vi "MonitorRheometer.vi"() -> ()   [LabVIEW 2017]
uses:
  ImageAcquisitionProgram/ImageAcquisitionLibrary/Acquisition/AcquireData.ctl
  ImageAcquisitionProgram/ImageAcquisitionLibrary/GlobalFrontPanelReferences.vi
  CoilsControl/FrontPanelReferences.vi
  AODControl/AODGlobals.vi
  AODControl/MessageQueue/QueueOperations/Enqueue Message (Single).vi
  ImageAcquisitionProgram/ImageAcquisitionLibrary/ImageAcquisitionLibrary.lvlib
  <vilib>/Analysis/NI_AAL_Geometry.lvlib
  <vilib>/gmath/NI_Gmath.lvlib
  CoilsControl/WaveformGenerator.lvlib
  AODControl/AODControl.lvlib
  AODControl/MessageQueue/MessageQueue.lvlib
panel:
  out "size(s)":i32
  out "r":dbl format="%.2f"
  out "logical OR":bool
  in  "stop":bool
  out "Tracking Data.Positions":dbl[][](array[numeric])
  out "XY Graph":cluster{dbl[], dbl[]}[](graph)
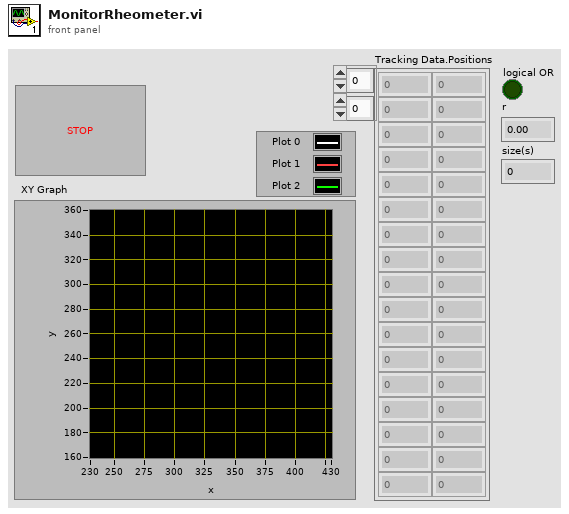
[diagram p1: front panel]
types:
  T1 = typedef "ImageAcquisitionLibrary.lvlib/AcquireData.ctl" = cluster{"Frame Data":cluster{"Image":u32[][], "Timestamp":timestamp, "Image Type":T2, "Dropped Frames":u32}, "Tracking Data":cluster{"Positions":dbl[][], "Timestamp":timestamp}, "Tracked?":bool}
  T2 = typedef "Image Type" = u32
  T3 = typedef "ImageAcquisitionLibrary.lvlib/References.ctl" = cluster{"Acquire":refnum<vi>, "Rec":refnum<vi>, "Tracking":refnum<vi>, "Settings":refnum<vi>, "Stop":refnum<vi>, "Initialized?":bool, "ImDisplay":refnum<vi>}
  T4 = typedef "WaveformGenerator.lvlib/WaveformGeneratorInterfaceRef.ctl" = cluster{"Waveform X":refnum<vi>, "Waveform Y":refnum<vi>, "Waveform Z":refnum<vi>, "Amplitude X":refnum<vi>, "Amplitude Y":refnum<vi>, "Amplitude Z":refnum<vi>, "Frequency X":refnum<vi>, "Frequency Y":refnum<vi>, "Frequency Z":refnum<vi>, "Phase X":refnum<vi>, "Phase Y":refnum<vi>, "Phase Z":refnum<vi>, "Offset X":refnum<vi>, "Offset Y":refnum<vi>, "Offset Z":refnum<vi>, "Stop":refnum<vi>, "On/Off":refnum<vi>, "Field^2":refnum<vi>}
  T5 = typedef "AODControl.lvlib/MessageQueue.lvlib/All Message Queues.ctl" = cluster{" AOD Interface":refnum<queue>}
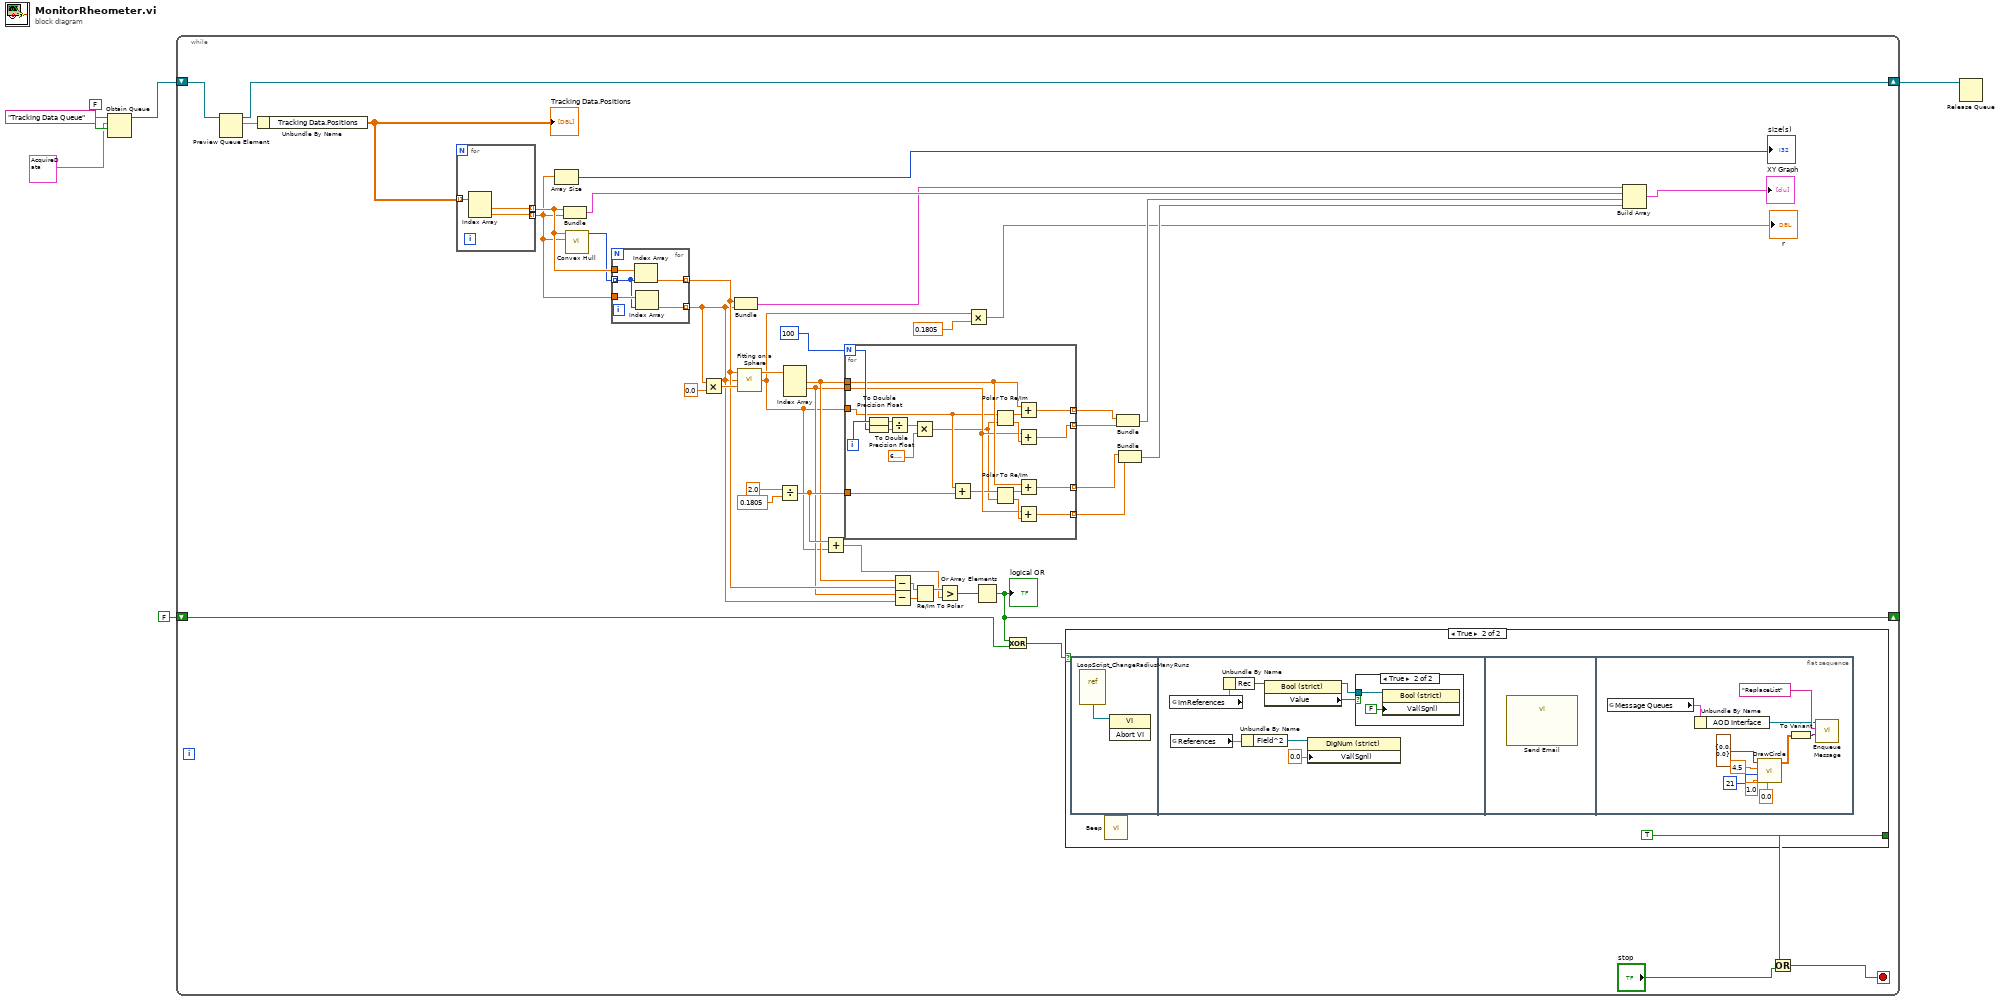
[diagram p0: block diagram]
diagram:
  n1 = Obtain Queue(name (unnamed)="Tracking Data Queue", element data type=T1 {"Frame Data"={"Image"=[], "Timestamp"=timestamp(0 s since 1904-01-01), "Image Type"=0, "Dropped Frames"=0}, "Tracking Data"={"Positions"=[], "Timestamp"=timestamp(0 s since 1904-01-01)}, "Tracked?"=FALSE} ("Acquired Data"), create if not found? (T)=FALSE) -> (queue out=w4:refnum<queue>)  [unwired: 2 in, 2 out]
  n2 = while {
    shift-right: [w45] -> w2
    shift-left: w4 -> [w48]
    shift-right: [w17] -> _
    shift-left: FALSE -> [w16]
    stop <- w9 stop-if-true
    n3 = Preview Queue Element(queue=w48) -> (queue out=w45:refnum<queue>, element=w47:T1)  [unwired: 2 in, 2 out]
    n4 = Unbundle By Name(w47) -> ("Tracking Data.Positions"=w46:dbl[][])
    "Tracking Data.Positions" <- w46
    n5 = for {
      tunnel: w46 -> [w97] mode=indexing
      tunnel: [w96] -> w44 mode=indexing
      tunnel: [w95] -> w11 mode=indexing
      n6 = Index Array(array=w97) -> (element #1=w96:dbl, element #2=w95:dbl)  [unwired: 2 in]
    }
    n7 = Array Size(array=w11) -> (size(s)=→"size(s)":i32)
    n8 = Bundle(w44, w11) -> (w41:cluster{dbl[], dbl[]})  [unwired: 1 in]
    n9 = call <vilib>:"Convex Hull.vi"("Y"=w11, "X"=w44) -> ("Convex Hull"=w43:i32[])  [unwired: 8 in, 1 out]
    n10 = for {
      tunnel: w44 -> [w94]
      tunnel: w11 -> [w93]
      tunnel: w43 -> [w92] mode=indexing
      tunnel: [w91] -> w19 mode=indexing
      tunnel: [w90] -> w21 mode=indexing
      n11 = Index Array(array=w94, index=w92) -> (element=w90:dbl)
      n12 = Index Array(array=w93, index=w92) -> (element=w91:dbl)
    }
    n13 = Multiply(x=w19, y=0.0 ("Numeric")) -> (x*y=w34:dbl[])
    n14 = Bundle(w21, w19) -> (w40:cluster{dbl[], dbl[]})  [unwired: 1 in]
    n15 = call <vilib>:"Fitting on a Sphere.vi"("Z"=w34, "Y"=w19, "X"=w21) -> ("r"=w12:dbl, "x0, y0, z0"=w38:dbl[])  [unwired: 1 out]
    n16 = Divide(x=2.0 ("y"), y=0.1805) -> (x/y=w27:dbl)
    n17 = Index Array(array=w38) -> (element #1=w22:dbl, element #2=w20:dbl)  [unwired: 3 in, 1 out]
    n18 = Add(x=w27, y=w12) -> (x+y=w23:dbl)
    n19 = for {
      N: 100 -> [w88]
      tunnel: w12 -> [w72]
      tunnel: w22 -> [w77]
      tunnel: w20 -> [w76]
      tunnel: [w81] -> w37 mode=indexing
      tunnel: [w80] -> w36 mode=indexing
      tunnel: [w74] -> w32 mode=indexing
      tunnel: [w73] -> w31 mode=indexing
      tunnel: w27 -> [w70]
      i -> [w89]
      n20 = To Double Precision Float(number=w89) -> (double precision float=w87:dbl)
      n21 = To Double Precision Float(number=w88) -> (double precision float=w86:dbl)
      n22 = Divide(x=w87, y=w86) -> (x/y=w84:dbl)
      n23 = Multiply(x=w84, y=6.283185307179586) -> (x*y=w71:dbl)
      n24 = Add(x=w72, y=w70) -> (x+y=w75:dbl)
      n25 = Polar To Re/Im(2:w71, 3:w72) -> (0:w83:dbl, 1:w82:dbl)
      n26 = Polar To Re/Im(2:w71, 3:w75) -> (0:w78:dbl, 1:w79:dbl)
      n27 = Add(x=w77, y=w82) -> (x+y=w81:dbl)
      n28 = Add(x=w76, y=w83) -> (x+y=w80:dbl)
      n29 = Add(x=w77, y=w79) -> (x+y=w74:dbl)
      n30 = Add(x=w76, y=w78) -> (x+y=w73:dbl)
    }
    n31 = Subtract(x=w22, y=w21) -> (x-y=w24:dbl[])
    n32 = Subtract(x=w20, y=w19) -> (x-y=w25:dbl[])
    n33 = Re/Im To Polar(2:w25, 3:w24) -> (1:w26:dbl[])  [unwired: 1 out]
    n34 = Greater?(x=w26, y=w23) -> (0:w18:bool[])
    n35 = Multiply(x=w12, y=0.1805) -> (x*y=→"r":dbl)
    n36 = Or Array Elements(Boolean array=w18) -> (logical OR=w17:bool)
    "logical OR" <- w17
    n37 = Exclusive Or(1:w16, 2:w17) -> (0:w15:bool)
    n38 = case shown="True" w15 {
      tunnel: [_ TRUE] -> w8
      frame False {
      }
      frame True {
        n39 = flat-sequence {
          frame #0 {
            n40 = vi-ref "LoopScript_ChangeRadiusManyRuns.vi"() -> (w50:refnum<vi>)
            n41 = invoke class="VI" method="Abort VI"(reference=w50) -> ()  [unwired: 2 in, 3 out]
          }
          frame #1 {
            n42 = global read "GlobalFrontPanelReferences.vi" "ImReferences"() -> (w57:T3)
            n43 = global read "FrontPanelReferences.vi" "References"() -> (w53:T4)
            n44 = Unbundle By Name(w57) -> ("Rec"=w56:refnum<vi>)
            n45 = Unbundle By Name(w53) -> ("Field^2"=w52:refnum<vi>)
            n46 = property class="Bool (strict)"(reference=w56) -> (reference out=w54:refnum<vi>, "Value"=w55:bool)  [unwired: 1 in, 1 out]
            n47 = property class="DigNum (strict)"(reference=w52, "Val(Sgnl)"=0.0 ("Value (Signaling)")) -> ()  [unwired: 1 in, 2 out]
            n48 = case shown="True" w55 {
              tunnel: w54 -> [_ w58]
              frame False {
              }
              frame True {
                n49 = property class="Bool (strict)"(reference=w58, "Val(Sgnl)"=FALSE ("Value (Signaling)")) -> ()  [unwired: 1 in, 2 out]
              }
            }
          }
          frame #2 {
            n50 = call "Send Email"() -> ()  [unwired: 11 in, 1 out]
          }
          frame #3 {
            n51 = global read "AODGlobals.vi" "Message Queues"() -> (w61:T5)
            n52 = Unbundle By Name(w61) -> ("AOD Interface"=w60:refnum<queue>)
            n53 = call "DrawCircle.vi"("Phase"=0.0, "Eccentricity"=1.0, "No Of Points"=21, "Radius"=4.5, "Center"=cluster{"X":dbl, "Y":dbl} {"X"=0.0, "Y"=0.0}) -> ("Array"=w69:dbl[][])  [unwired: 6 in]
            n54 = To Variant(anything=w69) -> (Variant=w68:variant)
            n55 = call-poly "Enqueue Message.vi"("Message Data"=w68, "Message"="ReplaceList", "Message Queue"=w60) -> ()  [unwired: 7 in, 2 out]
          }
        }
        n56 = call <vilib>:"Beep.vi"() -> ()  [unwired: 12 in]
      }
    }
    n57 = Bundle(w37, w36) -> (w35:cluster{dbl[], dbl[]})  [unwired: 1 in]
    n58 = Bundle(w32, w31) -> (w30:cluster{dbl[], dbl[]})  [unwired: 1 in]
    n59 = Build Array(w40, w41, w35, w30) -> (→"XY Graph":cluster{dbl[], dbl[]}[])
    n60 = Or(x=w8, y="stop") -> (x .or. y?=w9:bool)
  }
  n61 = Release Queue(queue=w2) -> ()  [unwired: 2 in, 3 out]
